vi "write to log file.vi"(0 "input":string, 1 "error in":errorcluster) -> (7 "log":string="2:40 PM\tStop DAQ...")   [LabVIEW 2019]
panel:
  in  "platform":u16
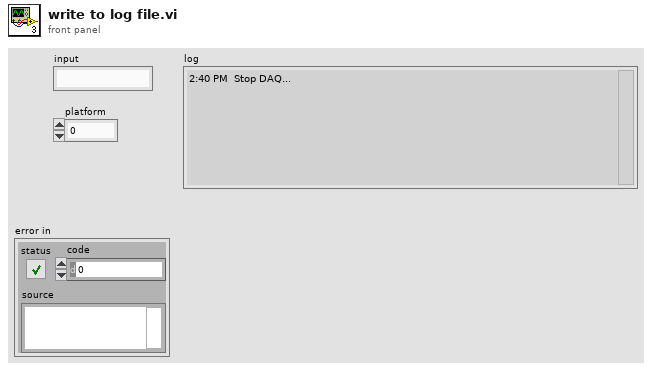
[diagram p1: front panel]
types:
  T1 = enum16{"open", "replace", "create", "open or create", "replace or create", "replace or create with confirmation"}
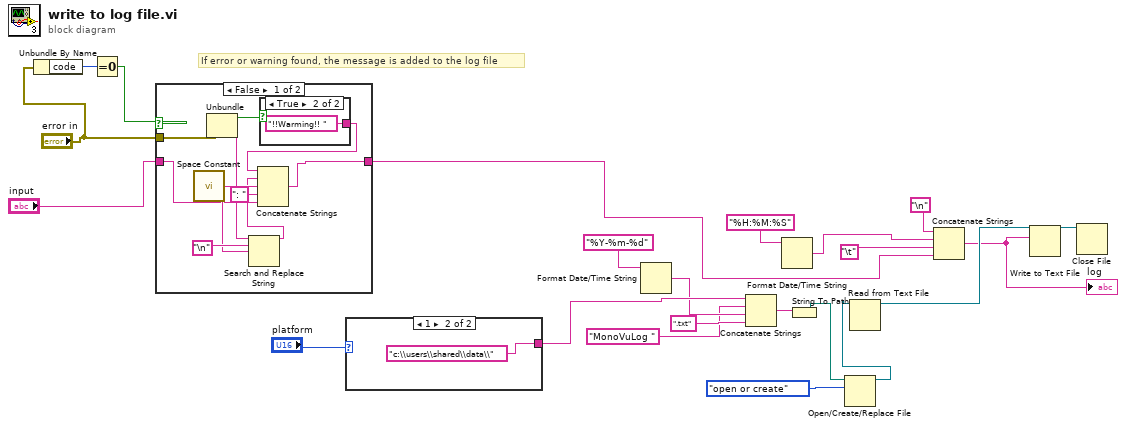
[diagram p0: block diagram]
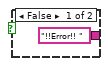
[diagram p2: hidden frame]
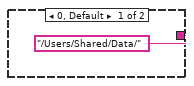
[diagram p4: hidden frame]
diagram:
  # "If error or warning found, the message is added to the log file"
  n1 = Unbundle By Name("error in") -> ("code"=w3:i32)
  n2 = Equal To 0?(x=w3) -> (x = 0?=w1:bool)
  n3 = case shown="False" w1 {
    tunnel: "input" -> [w24 w35]
    tunnel: [w32 w35] -> w4
    tunnel: "error in" -> [w31 _]
    frame False {
      n4 = call <vilib>:"Space Constant.vi"() -> ("String"=w26:string)
      n5 = Unbundle(w31) -> ("status"=w30:bool, "source"=w28:string)  [unwired: 1 out]
      n6 = Search and Replace String(input string=w28, search string="\n", replace string=w26) -> (result string=w25:string)  [unwired: 5 in, 3 out]
      n7 = case shown="True" w30 {
        tunnel: ["!!Error!! " ("string") "!!Warming!! " ("string")] -> w29
        frame False {
        }
        frame True {
        }
      }
      n8 = Concatenate Strings(w29, w25, w26, ": " ("string"), w24) -> (w32:string)
    }
    frame True {
    }
  }
  n9 = case shown="1" "platform" {
    tunnel: ["/Users/Shared/Data/" ("string") "c:\\users\\shared\\data\\" ("string")] -> w12
    frame 0, Default {
    }
    frame 1 {
    }
  }
  n10 = Format Date/Time String(time format string (%c)="%Y-%m-%d") -> (date/time string=w9:string)  [unwired: 2 in]
  n11 = Concatenate Strings(w12, "MonoVuLog " ("string"), w9, ".txt" ("string")) -> (w13:string)
  n12 = Format Date/Time String(time format string (%c)="%H:%M:%S") -> (date/time string=w22:string)  [unwired: 2 in]
  n13 = String To Path(string=w13) -> (path=w18:path)
  n14 = Open/Create/Replace File(file path (use dialog)=w18, operation (0:open)=T1."open or create") -> (refnum out=w20:refnum<file>)  [unwired: 4 in, 2 out]
  n15 = Read from Text File(file (use dialog)=w20) -> (refnum out=w17:refnum<file>)  [unwired: 3 in, 3 out]
  n16 = Concatenate Strings("\n", w22, "\t", w4) -> (w16:string)
  "log" <- w16
  n17 = Write to Text File(file (use dialog)=w17, text=w16) -> (refnum out=w21:refnum<file>)  [unwired: 2 in, 2 out]
  n18 = Close File(refnum=w21) -> ()  [unwired: 1 in, 2 out]
